vi "constructor.vi"(8 "error in (no error)":errorcluster, 10 "AnalyserType":string) -> (0 "error out":errorcluster, 3 "ImageAnalyser out":refnum<class "ImageAnalyser.lvclass">)   [LabVIEW 2011, in "Tools.lvlib" / "Imaging.lvlib" / "ImageAnalyser.lvclass"]
uses:
  ImageAnalyser.lvclass
  AbsorptionAnalyser/AbsorptionAnalyser.lvclass
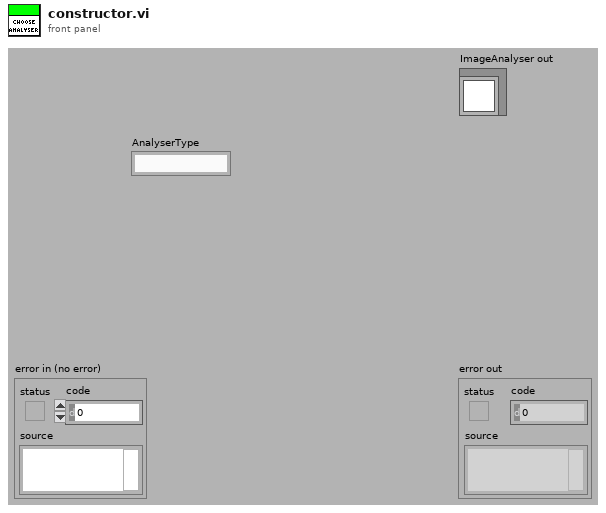
[diagram p1: front panel]
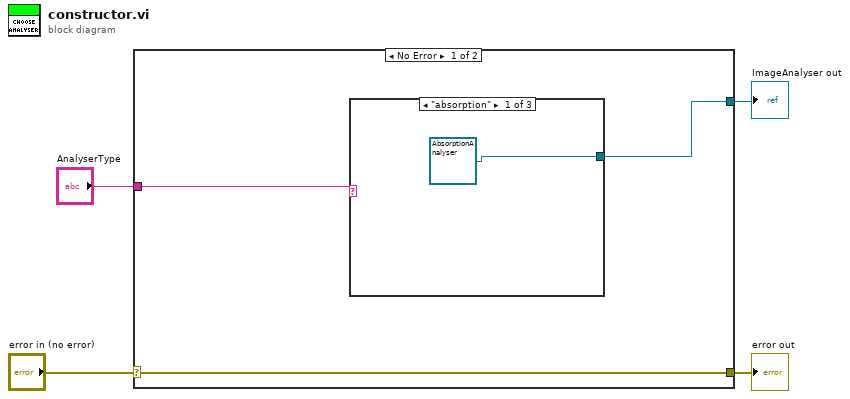
[diagram p0: block diagram]
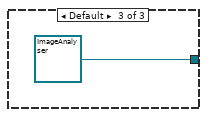
[diagram p3: hidden frame]
diagram:
  n1 = case shown="No Error" "error in (no error)" {
    selector: "error in (no error)" -> [w7 w10]
    tunnel: [w7 w10] -> w3
    tunnel: "AnalyserType" -> [w6 _]
    tunnel: [w5 _] -> w1
    frame No Error {
      n2 = case shown="\"absorption\"" w6 {
        tunnel: [refnum<class "AbsorptionAnalyser.lvclass"> refnum ("Tools.lvlib:Imaging.lvlib:AbsorptionAnalyser.lvclass") _ refnum<class "ImageAnalyser.lvclass"> refnum ("Tools.lvlib:Imaging.lvlib:ImageAnalyser.lvclass")] -> w5
        frame "absorption" {
        }
        frame "fluorescence " {
        }
        frame Default {
        }
      }
    }
    frame Error {
    }
  }
  "error out" <- w3
  "ImageAnalyser out" <- w1
